vi "Examples Images1.vi"() -> ()   [LabVIEW 2020, in "LcPictureBox.lvclass"]
uses:
  <userlib>/_LabVIEWCommon/LcPictureBox_class/LcPictureBox.lvclass
  <vilib>/picture/picture.llb/imagedata.ctl
  <userlib>/_LabVIEWCommon/LcPictureBox_class/SmoothingMode.ctl
  System.Windows.Forms
panel:
  out "Numeric":i32
  out "Error Out":errorcluster
  in  "PictureBox":refnum<k24>(container)
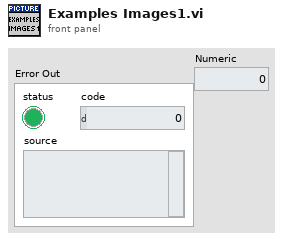
[diagram p1: front panel]
types:
  T1 = typedef "imagedata.ctl" = cluster{"image type":i32, "image depth":i32, "image":u8[], "mask":u8[], "colors":u32[], "Rectangle":cluster{"left":i16, "top":i16, "right":i16, "bottom":i16}}
  T2 = typedef "LcPictureBox.lvclass/SmoothingMode.ctl" = enum16{"None", "HighSpeed", "HighQuality", "AntiAlias"}
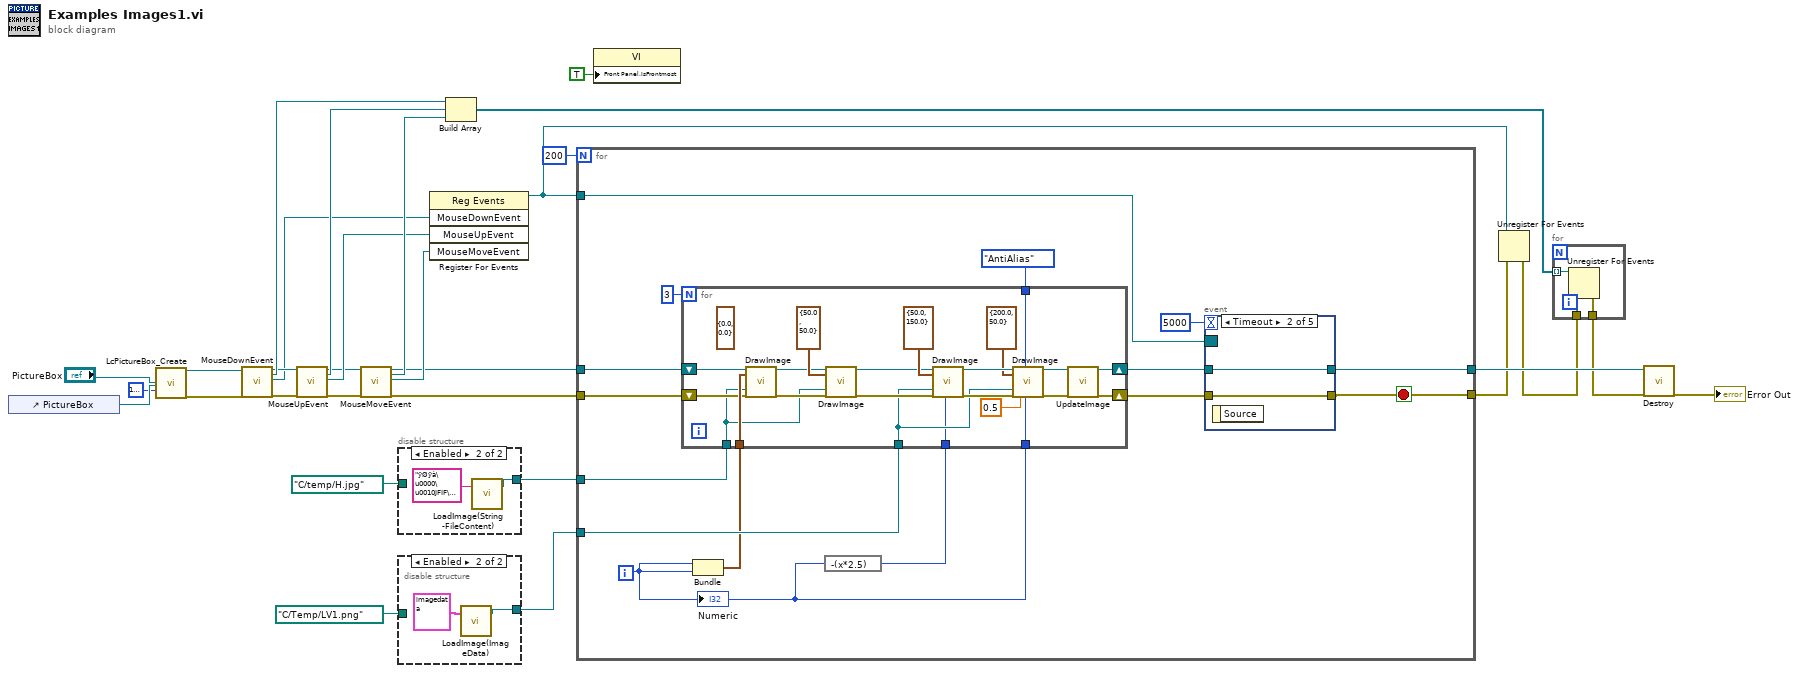
[diagram p0: block diagram]
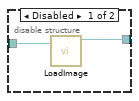
[diagram p2: hidden frame]
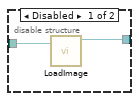
[diagram p3: hidden frame]
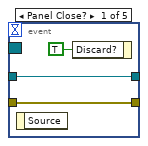
[diagram p4: hidden frame]
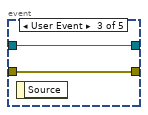
[diagram p5: hidden frame]
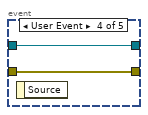
[diagram p6: hidden frame]
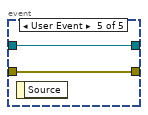
[diagram p7: hidden frame]
diagram:
  n1 = control-ref of="PictureBox"() -> (w24:refnum<vi>)
  n2 = call <userlib>:"LcPictureBox_Create.vi"("PictureBox"="PictureBox", "PictureBoxActiveXReference"=w24, "BgColor(None)"=u32 16777216) -> ("reference out"=w9:refnum<class "LcPictureBox.lvclass">, "Error Out"=w8:errorcluster)  [unwired: 14 in, 1 out]
  n3 = call-dynamic "MouseDownEvent.vi"("reference in"=w9, "error in (no error)"=w8) -> ("reference out"=w11:refnum<class "LcPictureBox.lvclass">, "Event Callback Refnum"=w16:refnum<k27>, "MouseDownEvent"=w10:refnum<user-event>, "error out"=w13:errorcluster)  [unwired: 14 in]
  n4 = call-dynamic "MouseUpEvent.vi"("reference in"=w11, "error in (no error)"=w13) -> ("reference out"=w12:refnum<class "LcPictureBox.lvclass">, "Event Callback Refnum"=w17:refnum<k27>, "MouseUpEvent"=w14:refnum<user-event>, "error out"=w15:errorcluster)  [unwired: 14 in]
  n5 = call-dynamic "MouseMoveEvent.vi"("reference in"=w12, "error in (no error)"=w15) -> ("reference out"=w7:refnum<class "LcPictureBox.lvclass">, "Event Callback Refnum"=w18:refnum<k27>, "MouseMoveEvent"=w19:refnum<user-event>, "error out"=w6:errorcluster)  [unwired: 14 in]
  n6 = disable-structure shown="Enabled" {
    disable-tunnel: path "C:/temp/H.jpg" ("Filename") -> [w32 _]
    disable-tunnel: [w31 w34] -> w28
    frame Disabled {
      n7 = call <userlib>:"LoadImage.vi"("ImageFile"=w32) -> ("ImageOut"=w31:refnum<k24>)  [unwired: 16 in, 2 out]
    }
    frame Enabled {
      n8 = call <userlib>:"LoadImage(String-FileContent).vi"("ImageFileContent"="ÿØÿà\u0000\u0010JFIF\u0000\u0001\u0001\u0000\u0000\u0001\u0000\u0001\u0000\u0000ÿÛ\u0000\u0000\t\u0006\u0007\r\u000f\r\r\r\r\r\r\r\r\r\r\u000f\r\r\r\r\r\u000f\r\r\r\r\u0015\u0011\u0016\u0016\u0015\u0011\u0015\u0015\u0018(( \u0018\u001a%\u001b\u0015\u0015!1!%)+...\u0017\u001f383,7(1:.\u0001\n\n\n\u000e\r\u000e\u0015\u0010\u0010\u0015/\u001d\u0016\u0019++-7+---+++-++++++++-7++-+--+---+-++++----++7+-.++ÿÀ\u0000\u0011\b\u0000á\u0000á\u0003\u0001\"\u0000\u0002\u0011\u0001\u0003\u0011\u0001ÿÄ\u0000\u001c\u0000\u0000\u0002\u0001\u0005\u0001\u0000\u0000\u0000\u0000\u0000\u0000\u0000\u0000\u0000\u0000\u0000\u0000\u0002\u0001\u0003\u0004\u0005\u0006\u0007\bÿÄ\u0000I\u0010\u0000\u0001\u0003\u0001\u0001\u0006\u0010\n\t\u0005\u0001\u0001\u0000\u0000\u0000\u0000\u0000\u0001\u0002\u0011\u0003\u0004\u0005\u0006\u0012Rrs\u0007\u0013\u0014\u0016!135S±²ÁÑ\u0017\"#24AQqt\b%BCUa¡¤ã\u0015Tbð¢áÿÄ\u0000\u0018\u0001\u0001\u0000\u0003\u0001\u0000\u0000\u0000\u0000\u0000\u0000\u0000\u0000\u0000\u0000\u0000\u0000\u0000\u0001\u0002\u0003\u0004ÿÄ\u0000 \u0011\u0001\u0000\u0002\u0002\u0002\u0002\u0003\u0001\u0000\u0000\u0000\u0000\u0000\u0000\u0000\u0000\u0000\u0001\u0002\u00031\u0011\u0012\u00132AQR!ÿÚ\u0000\f\u0003\u0001\u0000\u0002\u0011\u0003\u0011\u0000?\u0000î ª\n¦\u0006ê]*¨k2aUw%õ¹ËêA3ÀÉZ®\u001a~sÑ>f6¥ôÙQc\r¼dÙ®\u001d\u0016Ãë®¨«¶ªÿ\u00001\u0017òoye*hÚLDö#Za9£â9[«\u0017®Ë.;xÃ]\\vñl\u0016pmâ@Áo\u0006Þ$\u001eiüXvYqÛÆ\u001aì²ã·Ë`·o\u0012\u0006\u000bx6ñ óOäêÄë²ËÞ0×e\u001d¼f[\u0005¼\u001by(\u0018-àÛÄÍ?«\u0013®Ë.;xÃ]\\vñl\u0016ðmâ@Áo\u0006Þ$\u001eiüXvYqÛÆ\u001aì²ã·Ë`·o\u0012\u0006\u000bx6òPy§òubuÙeÇo\u0018k²ËÞ3-Þ\r¼\f\u0016ðm..." ("Display")) -> ("ImageOut"=w34:refnum<k24>)  [unwired: 16 in, 2 out]
    }
  }
  n9 = disable-structure shown="Enabled" {
    disable-tunnel: path "C:/Temp/LV1.png" ("Filename") -> [w36 _]
    disable-tunnel: [w35 w38] -> w27
    frame Disabled {
      n10 = call <userlib>:"LoadImage.vi"("ImageFile"=w36) -> ("ImageOut"=w35:refnum<k24>)  [unwired: 16 in, 2 out]
    }
    frame Enabled {
      n11 = call <userlib>:"LoadImage(ImageData).vi"("image data"=T1 {"image type"=0, "image depth"=8, "image"=array[50624 elements], "mask"=[], "colors"=[16767516, 16777215, 0, 16766720, 16776692, 16767232, 16769309, 16768284, 16768797, 10586386, 8482318, 5589257, 13216790, 15649818, 16769821, 16767509, 3813638, 12361749, 16775651, 16770159, 16772255, 16773042, 16776695, 16768578, 16776174, 16775131, 16773304, 16774345, 16774868, 16770426, 16771734, 16771470, 16770688, 16769375, 16768843, 16772521, 16773824, 16768583, 16769108, 16768050, 16771737, 16770163, 16775649, 16175899, 10126097, 7824653, 16768312, 16769638, 7101452, 2564356, 4865800, 0, 0, 0, 0, 0, 0, 0, 0, 0, 0, 0, 0, 0, 0, 0, 0, 0, 0, 0, 0, 0, 0, 0, 0, 0, 0, 0, 0, 0, 0, 0, 0, 0, 0, 0, 0, 0, 0, 0, 0, 0, 0, 0, 0, 0, 0, 0, 0, 0, 0, 0, 0, 0, 0, 0, 0, 0, 0, 0, 0, 0, 0, 0, 0, 0, 0, 0, 0, 0, 0, 0, 0, 0, 0, 0, 0, 0, 0, 0, 0, 0, 0, 0, 0, 0, 0, 0, 0, 0, 0, 0, 0, 0, 0, 0, 0, 0, 0, 0, 0, 0, 0, 0, 0, 0, 0, 0, 0, 0, 0, 0, 0, 0, 0, 0, 0, 0, 0, 0, 0, 0, 0, 0, 0, 0, 0, 0, 0, 0, 0, 0, 0, 0, 0, 0, 0, 0, 0, 0, 0, 0, 0, 0, 0, 0, 0, 0, 0, 0, 0, 0, 0, 0, 0, 0, 0, 0, 0, 0, 0, 0, 0, 0, 0, 0, 0, 0, 0, 0, 0, 0, 0, 0, 0, 0, 0, 0, 0, 0, 0, 0, 0, 0, 0, 0, 0, 0, 0, 0, 0, 0, 0, 0, 0, 0, 0, 0, 0, 0, 0, 0, 0, 0, 0, 0], "Rectangle"={"left"=0, "top"=0, "right"=223, "bottom"=226}}) -> ("ImageOut"=w38:refnum<k24>)  [unwired: 16 in, 2 out]
    }
  }
  n12 = register-events(w10, w14, w19) -> (reference out=w1:refnum<event-registration>)  [unwired: 2 in, 1 out]
  n13 = Build Array(w16, w17, w18) -> (w5:refnum<k27>[])
  n14 = for {
    N: 200 -> [_]
    tunnel: w27 -> [w53]
    tunnel: [w41] -> w3
    tunnel: w28 -> [w50]
    tunnel: [w45] -> w22
    tunnel: w1 -> [w44]
    tunnel: w7 -> [w43]
    tunnel: w6 -> [w42]
    i -> [w39]
    stop <- w41 stop-if-true
    n15 = Bundle(w39, w39) -> (w47:cluster{i32, i32})  [unwired: 1 in]
    n16 = expression code="-(x*2.5)"(w39) -> (w40:i32)
    n17 = for {
      N: 3 -> [_]
      tunnel: w53 -> [w56]
      tunnel: w50 -> [w57]
      tunnel: SmoothingMode."AntiAlias" ("SmoothingMode") -> [w61]
      tunnel: w47 -> [w60]
      shift-right: [w65] -> w51
      shift-left: w43 -> [w59]
      shift-right: [w67] -> w52
      shift-left: w42 -> [w58]
      tunnel: w39 -> [w55]
      tunnel: w40 -> [w54]
      (unwired) cluster{"x":sgl, "y":sgl} {"x"=0.0, "y"=0.0} ("UpperLeftCorner")
      n18 = call-dynamic "DrawImage.vi"("reference in"=w59, "UpperLeftCorner(0,0)"=w60, "Image"=w57, "Error In"=w58) -> ("reference out"=w64:refnum<class "LcPictureBox.lvclass">, "Error Out"=w63:errorcluster)  [unwired: 13 in, 1 out]
      n19 = call-dynamic "DrawImage.vi"("reference in"=w64, "UpperLeftCorner(0,0)"=cluster{"x":sgl, "y":sgl} {"x"=50.0, "y"=50.0} ("UpperLeftCorner"), "Image"=w57, "Error In"=w63) -> ("reference out"=w72:refnum<class "LcPictureBox.lvclass">, "Error Out"=w73:errorcluster)  [unwired: 13 in, 1 out]
      n20 = call-dynamic "DrawImage.vi"("reference in"=w72, "UpperLeftCorner(0,0)"=cluster{"x":sgl, "y":sgl} {"x"=50.0, "y"=150.0} ("UpperLeftCorner"), "Image"=w56, "Error In"=w73, "Rotation(Deg)"=w54) -> ("reference out"=w71:refnum<class "LcPictureBox.lvclass">, "Error Out"=w70:errorcluster)  [unwired: 12 in, 1 out]
      n21 = call-dynamic "DrawImage.vi"("reference in"=w71, "UpperLeftCorner(0,0)"=cluster{"x":sgl, "y":sgl} {"x"=200.0, "y"=50.0} ("UpperLeftCorner"), "Image"=w56, "Error In"=w70, "ScaleFactor(1)"=0.5, "SmoothingMode(AntiAlias)"=w61, "Rotation(Deg)"=w55) -> ("reference out"=w66:refnum<class "LcPictureBox.lvclass">, "Error Out"=w68:errorcluster)  [unwired: 10 in, 1 out]
      n22 = call-dynamic "UpdateImage.vi"("reference in"=w66, "Error In"=w68) -> ("reference out"=w65:refnum<class "LcPictureBox.lvclass">, "Error Out"=w67:errorcluster)  [unwired: 14 in, 2 out]
    }
    n23 = event shown="[1] Timeout" {
      selector: w44 -> [_ _ _ _ _]
      dyn-events: _ -> [_ _ _ _ _]
      timeout: 5000 -> [_ _ _ _ _]
      tunnel: w52 -> [w78 w79 w81 w83 w85]
      tunnel: [w78 w79 w81 w83 w85] -> w41
      tunnel: w51 -> [w76 w80 w82 w84 w86]
      tunnel: [w76 w80 w82 w84 w86] -> w45
      event Panel Close? {
        n24 = event-data() -> ()  [unwired: 1 in, 1 out]
        n25 = event-data("Discard?"=TRUE) -> ()  [unwired: 1 in, 1 out]
      }
      event Timeout {
        n26 = event-data() -> ()  [unwired: 1 in, 1 out]
      }
      event User Event {
        n27 = event-data() -> ()  [unwired: 1 in, 1 out]
      }
      event User Event {
        n28 = event-data() -> ()  [unwired: 1 in, 1 out]
      }
      event User Event {
        n29 = event-data() -> ()  [unwired: 1 in, 1 out]
      }
    }
    "Numeric" <- w39
  }
  n30 = property class="VI"("Front Panel.IsFrontmost"=TRUE ("Front Panel Window:Is Frontmost")) -> ()  [unwired: 2 in, 2 out]
  n31 = Unregister For Events(event registration refnum=w1, error in=w3) -> (error out=w2:errorcluster)
  n32 = for {
    tunnel: w2 -> [w89]
    tunnel: w5 -> [w88] mode=indexing
    tunnel: [w87] -> w4
    n33 = Unregister For Events(event registration refnum=w88, error in=w89) -> (error out=w87:errorcluster)
  }
  n34 = call-dynamic "Destroy.vi"("reference in"=w22, "Error In"=w4) -> ("Error Out"=→"Error Out":errorcluster)  [unwired: 16 in, 1 out]
